vi "TS_Request Multiple DTCs.vi"(8 "error in":errorcluster, 9 "Command":string, 10 "addresses":T1[](array[typedef]) {"Name" format="%.0x"}, 11 "internal data":T2={"J1939 XNET Settings"={"XNET Database"="", "XNET Cluster"="", "CAN port"="", "Baud rate [Bd]"=0, "J1939 Network Address"=0, "Name"=0, "Termination"=0}, "j1939 queues"={"Processed Outgoing"=refnum, "Process Outgoing"=refnum, "stop notifier"=refnum, "error queue"=refnum, "active dtc"=refnum, "processed inc"=refnum}, "fgv references"={"BAM Buffer"=refnum, "CM Buffer"=refnum, "CM Gen"=refnum, "BAM Gen"=refnum, "Address Claims"=refnum, "RQST"=refnum, "scaling lut"=refnum, "data lut"=refnum, "cyclic scheduler"=refnum}, "frame in"="", "frame out"="", "timing"={"tb to j1939 queue timeout"=100, "j1939 to tb queue timeout"=100, "dtc loop period (ms)"=100, "CAN in loop period (ms)"=100, "process incoming queue timeout (ms)"=100, "Outgoing Write Decimation"=0, "process outgoing loop rate (ms)"=0, "periodic outgoing queue timeout (ms)"=10, "CAN out queue timeout (ms)"=100}}) -> (0 "error out":errorcluster, 1 "Responses":T15[](array[typedef]))   [LabVIEW 2013, in "J1939.lvlib"]
uses:
  J1939.lvlib
  API Types/Convert DTCs Cluster.ctl
  API Types/Internal Data.ctl
  API Types/XNET Settings.ctl
  API Types/Setup Information Cluster.ctl
  API Types/CAN Outgoing Message Cluster.ctl
  <vilib>/xnet/xnet.llb/XNET Frame CAN.ctl
  <vilib>/xnet/xnet.llb/XNET Frame Type CAN.ctl
  TP/TP List References.ctl
  BAM/BAM Buffer Connections List_Ref.ctl
  Connection Mode/Connection Mode Generation Connection Ref.ctl
  BAM/BAM Generation Connections List_Ref.ctl
  LUTs/J1939 Address Table Reference.ctl
  RQST/RQST Lookup Table Reference.ctl
  LUTs/J1939 Conversion Lookup Table Reference.ctl
  LUTs/J1939 Data Lookup Table Reference.ctl
  LUTs/Cyclic Frame Scheduler Lut Reference.ctl
  Configuration/TypeDefs/timing configuration.ctl
  LUTs/J1939 Address Lookup Table Data.ctl
  API Types/WS Error Types.ctl
  API Types/WS_Request Message.ctl
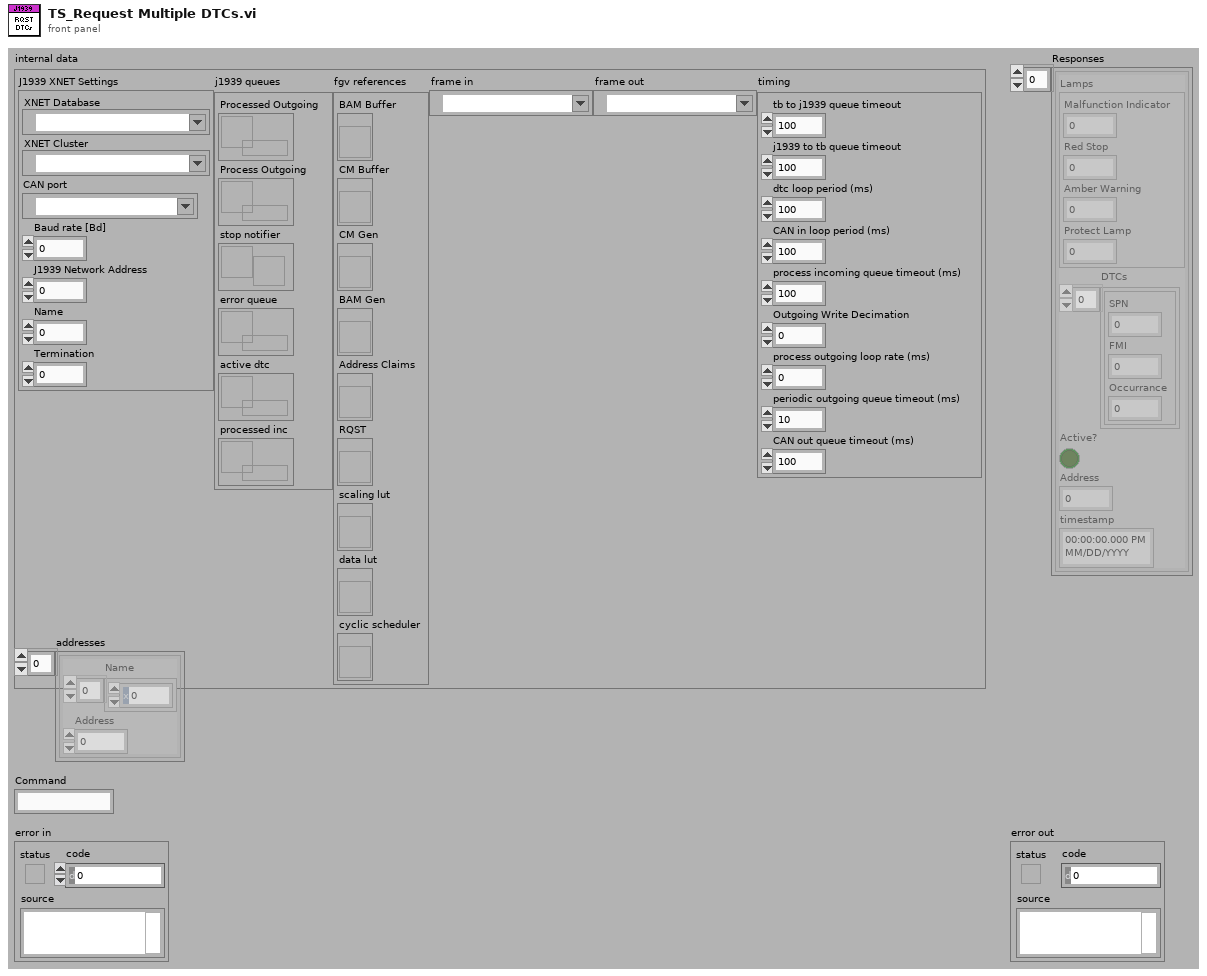
[diagram p1: front panel]
types:
  T1 = typedef "J1939.lvlib/J1939 Address Lookup Table Data.ctl" = cluster{"Name":u8[], "Address":u8}
  T2 = typedef "J1939.lvlib/Internal Data.ctl" = cluster{"J1939 XNET Settings":T3, "j1939 queues":T4, "fgv references":T5, "frame in":refnum<k21>, "frame out":refnum<k21>, "timing":T14}
  T3 = typedef "J1939.lvlib/XNET settings.ctl" = cluster{"XNET Database":refnum<k21>, "XNET Cluster":refnum<k21>, "CAN port":refnum<k21>, "Baud rate [Bd]":u32, "J1939 Network Address":u8, "Name":u64, "Termination":u32}
  T4 = typedef "J1939.lvlib/Setup Information Cluster.ctl" = cluster{"Processed Outgoing":refnum<queue>, "Process Outgoing":refnum<queue>, "stop notifier":refnum<notifier>, "error queue":refnum<queue>, "active dtc":refnum<queue>, "processed inc":refnum<queue>}
  T5 = typedef "J1939.lvlib/TP List References.ctl" = cluster{"BAM Buffer":T6, "CM Buffer":T6, "CM Gen":T7, "BAM Gen":T8, "Address Claims":T9, "RQST":T10, "scaling lut":T11, "data lut":T12, "cyclic scheduler":T13}
  T6 = typedef "J1939.lvlib/BAM Buffer Connections List_Ref.ctl" = refnum<vi>
  T7 = typedef "J1939.lvlib/Connection Mode Generation Connection Ref.ctl" = refnum<vi>
  T8 = typedef "J1939.lvlib/BAM Generation Connections List_Ref.ctl" = refnum<vi>
  T9 = typedef "J1939.lvlib/J1939 Address Table Reference.ctl" = refnum<vi>
  T10 = typedef "J1939.lvlib/RQST Lookup Table Reference.ctl" = refnum<vi>
  T11 = typedef "J1939.lvlib/J1939 Conversion Lookup Table Reference.ctl" = refnum<vi>
  T12 = typedef "J1939.lvlib/J1939 Data Lookup Table Reference.ctl" = refnum<vi>
  T13 = typedef "J1939.lvlib/cyclic frame scheduler lut reference.ctl" = refnum<vi>
  T14 = typedef "J1939.lvlib/timing configuration.ctl" = cluster{"tb to j1939 queue timeout":i32, "j1939 to tb queue timeout":i32, "dtc loop period (ms)":i32, "CAN in loop period (ms)":i32, "process incoming queue timeout (ms)":i32, "Outgoing Write Decimation":u32, "process outgoing loop rate (ms)":i32, "periodic outgoing queue timeout (ms)":i32, "CAN out queue timeout (ms)":i32}
  T15 = typedef "J1939.lvlib/Convert DTCs Cluster.ctl" = cluster{"Lamps":cluster{"Malfunction Indicator":u8, "Red Stop":u8, "Amber Warning":u8, "Protect Lamp":u8}, "DTCs":cluster{"SPN":u32, "FMI":u8, "Occurrance":u8}[], "Active?":bool, "Address":u8, "timestamp":timestamp}
  T16 = typedef "J1939.lvlib/WS Error Types.ctl" = enum16{"Request", "RAW Generation", "Clear Active DTCs", "Clear Previous DTCs", "Addresses", "TLAs", "Get Active DTCs", "Get Previous DTCs"}
  T17 = typedef "J1939.lvlib/WS_Request Message.ctl" = cluster{"PGN":u32, "DA":u8, "Ignore Response":bool}
  T18 = typedef "XNET Frame CAN.ctl" = cluster{"timestamp":timestamp, "payload":u8[], "identifier":u32, "type":T19, "extended?":bool, "echo?":bool}
  T19 = typedef "XNET Frame Type CAN.ctl" = u8
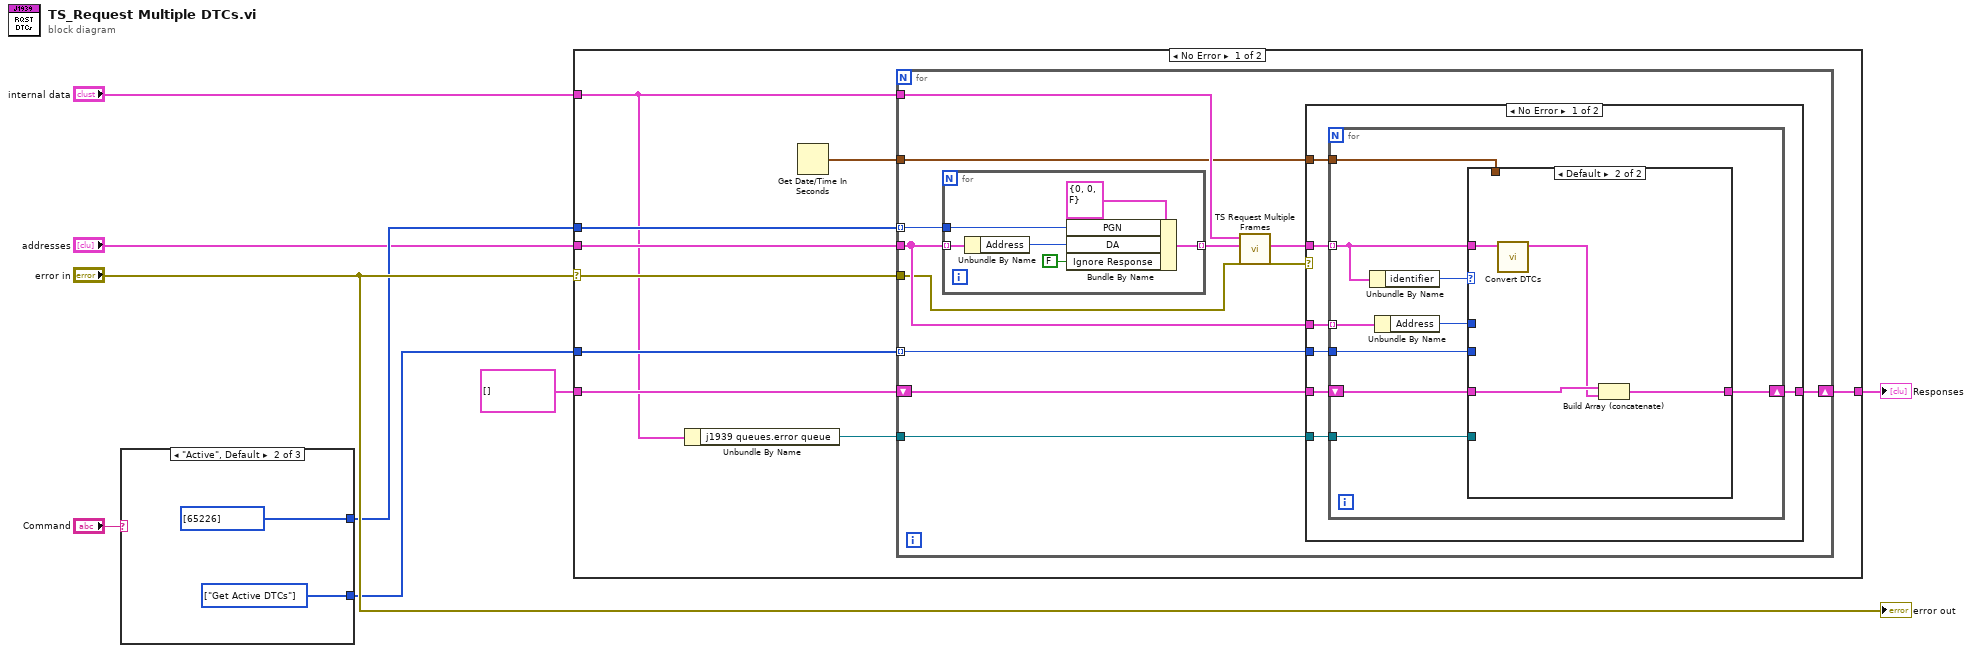
[diagram p0: block diagram]
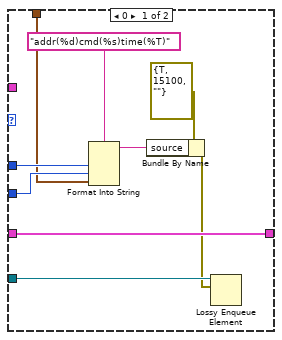
[diagram p2: hidden frame]
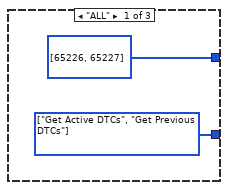
[diagram p5: hidden frame]
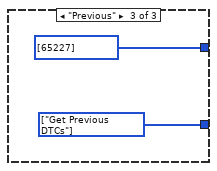
[diagram p6: hidden frame]
diagram:
  n1 = case shown="\"Active\", Default" "Command" {
    tunnel: [u32[] [65226, 65227] u32[] [65226] u32[] [65227]] -> w6
    tunnel: [w9 w11 w13] -> w5
    frame "ALL" {
      w9 = T16[] [enum."Get Active DTCs", enum."Get Previous DTCs"] items=["Request", "RAW Generation", "Clear Active DTCs", "Clear Previous DTCs", "Addresses", "TLAs", "Get Active DTCs", "Get Previous DTCs"]
    }
    frame "Active", Default {
      w11 = T16[] [enum."Get Active DTCs"] items=["Request", "RAW Generation", "Clear Active DTCs", "Clear Previous DTCs", "Addresses", "TLAs", "Get Active DTCs", "Get Previous DTCs"]
    }
    frame "Previous" {
      w13 = T16[] [enum."Get Previous DTCs"] items=["Request", "RAW Generation", "Clear Active DTCs", "Clear Previous DTCs", "Addresses", "TLAs", "Get Active DTCs", "Get Previous DTCs"]
    }
  }
  n2 = case shown="No Error" "error in" {
    selector: "error in" -> [w18 _]
    tunnel: "internal data" -> [w16 _]
    tunnel: "addresses" -> [w23 _]
    tunnel: w6 -> [w22 _]
    tunnel: w5 -> [w21 _]
    tunnel: T15[] [] -> [w20 w72]
    tunnel: [w19 w72] -> w3
    frame No Error {
      n3 = Unbundle By Name(w16) -> ("j1939 queues.error queue"=w15:refnum<queue>)
      n4 = Get Date/Time In Seconds() -> (seconds since 1Jan1904=w17:timestamp)
      n5 = for {
        tunnel: w23 -> [w31]
        tunnel: w22 -> [w30] mode=indexing
        tunnel: w21 -> [w29] mode=indexing
        shift-right: [w27] -> w19
        shift-left: w20 -> [w28]
        tunnel: w18 -> [w26]
        tunnel: w16 -> [w34]
        tunnel: w17 -> [w25]
        tunnel: w15 -> [w24]
        n6 = for {
          tunnel: w31 -> [w70] mode=indexing
          tunnel: [w67] -> w35 mode=indexing
          tunnel: w30 -> [w66]
          n7 = Unbundle By Name(w70) -> ("Address"=w69:u8)
          n8 = Bundle By Name(cluster=T17 {"PGN"=0, "DA"=0, "Ignore Response"=FALSE} ("Cluster"), "PGN"=w66, "DA"=w69, "Ignore Response"=FALSE) -> (w67:T17)
        }
        n9 = call "TS Request Multiple Frames.vi"("error in"=w26, "Requests"=w35, "internal data"=w34) -> ("error out"=w33:errorcluster, "Response Frames"=w32:T18[])  [unwired: 7 in]
        n10 = case shown="No Error" w33 {
          tunnel: w32 -> [w42 _]
          tunnel: w28 -> [w41 w65]
          tunnel: w31 -> [w40 _]
          tunnel: w29 -> [w39 _]
          tunnel: [w38 w65] -> w27
          tunnel: w25 -> [w37 _]
          tunnel: w24 -> [w36 _]
          frame No Error {
            n11 = for {
              tunnel: w42 -> [w50] mode=indexing
              shift-right: [w48] -> w38
              shift-left: w41 -> [w49]
              tunnel: w40 -> [w47] mode=indexing
              tunnel: w39 -> [w45]
              tunnel: w37 -> [w43]
              tunnel: w36 -> [w44]
              n12 = Unbundle By Name(w50) -> ("identifier"=w51:u32)
              n13 = Unbundle By Name(w47) -> ("Address"=w46:u8)
              n14 = case shown="Default" w51 {
                tunnel: w50 -> [_ w64]
                tunnel: w49 -> [w60 w63]
                tunnel: [w60 w61] -> w48
                tunnel: w45 -> [w54 _]
                tunnel: w46 -> [w58 _]
                tunnel: w44 -> [w59 _]
                tunnel: w43 -> [w53 _]
                frame 0 {
                  n15 = Format Into String(format string="addr(%d)cmd(%s)time(%T)", w58, w54, w53) -> (resulting string=w56:string)  [unwired: 2 in, 1 out]
                  n16 = Bundle By Name(cluster=errorcluster {"status"=TRUE, "code"=15100, "source"=""} ("error IO"), "source"=w56) -> (w55:errorcluster)
                  n17 = Lossy Enqueue Element(queue=w59, element=w55) -> ()  [unwired: 1 in, 4 out]
                }
                frame Default {
                  n18 = call "Convert DTCs.vi"("value"=w64) -> ("Cluster"=w62:T15)  [unwired: 10 in]
                  n19 = Build Array (concatenate)(w63, w62) -> (w61:T15[])
                }
              }
            }
          }
          frame Error {
          }
        }
      }
    }
    frame Error {
    }
  }
  "Responses" <- w3
  "error out" <- "error in"
